vi "Position Map or Images Button.vi"(8 "error in (no error)":errorcluster, 11 "Button Ref":refnum<vi>) -> (0 "error out":errorcluster)   [LabVIEW 2014]
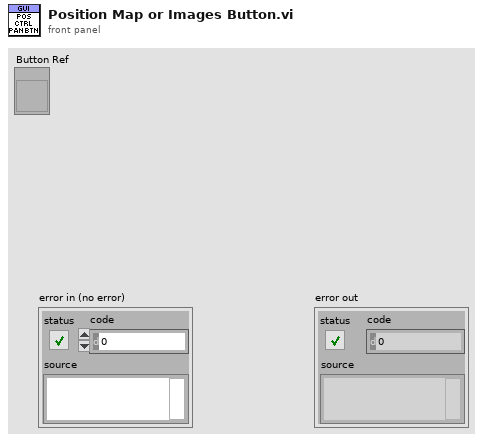
[diagram p1: front panel]
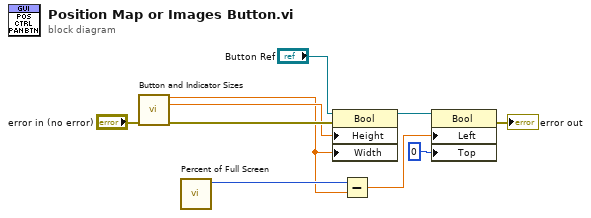
[diagram p0: block diagram]
diagram:
  n1 = call "Button and Indicator Sizes.vi"("error in (no error)"="error in (no error)") -> ("Button Width"=w3:dbl, "Button Height"=w7:dbl, "error out"=w9:errorcluster)  [unwired: 10 in, 2 out]
  n2 = call "Percent of Full Screen.vi"() -> ("Right"=w4:i16)  [unwired: 9 in, 2 out]
  n3 = property class="Bool"(reference="Button Ref", error in=w9, "Height"=w7, "Width"=w3) -> (reference out=w6:refnum<vi>)  [unwired: 1 out]
  n4 = Subtract(x=w4, y=w3) -> (x-y=w2:dbl)
  n5 = property class="Bool"(reference=w6, "Left"=w2, "Top"=0 ("Position:Top")) -> (error out=→"error out":errorcluster)  [unwired: 1 in, 1 out]
